vi "S4 Step Run For Scan.vi"(8 "error in (no error)":errorcluster) -> (0 "error out":errorcluster)   [LabVIEW 2019]
uses:
  NG Pick/NG Pick.lvclass
  Ctrl/Station Action.ctl
  Ctrl/ProjectStepSelect.ctl
  Ctrl/StationCmdSelect.ctl
  Ctrl/Auto Inspection Station Name2.ctl
  Ctrl/Auto Inspection Data Name.ctl
  Ctrl/S2 Station IO.ctl
  Global/Process Global.vi
  LineScan/LineScan.lvclass
  Ctrl/MeasureDisplayTab.ctl
  Ctrl/Table Save.ctl
  LLB/Commonly VI/Main Glb.vi
  LLB/Commonly VI.lvlib
panel:
  in  "Table Control":string[][](table)=[["PCBA BARCODE", ""], ["硬體(Tool初始化)", ""], ["company(Tool初始化)", ""], ["耗電流 uA(電流表)", "T"], ["電池負載電壓", "T"], ["晶片ID(Tool FORMAT)", "F"], ["雷雕ID(TOOl scan、藍芽接收器)", "S"], ["Format(Tool FORMAT)", "F"], ["Programe(Tool Programe)", "P"]]
  out "Numeric":dbl
  out "subarray":string[](array[string])
  out "S2 receive":string
  out "Blue Scan2 receive":string
  out "S1 receive":string
  out "S1 ToolStringOut":string
  out "S1 ChkSum":string
  out "Blue Scan receive":string
  out "Array":string[](array[string])
  out "present":i32
  out "Retry":i32
  out "Act Step":i32
  out "retry次數":string[](array[string])
  out "CurrentCmd":string
  out "Station Out":T1=enum."ImformOut"
  out "NG Pick out":refnum<class "NG Pick.lvclass">
  in  "NG Pick in":refnum<class "NG Pick.lvclass">
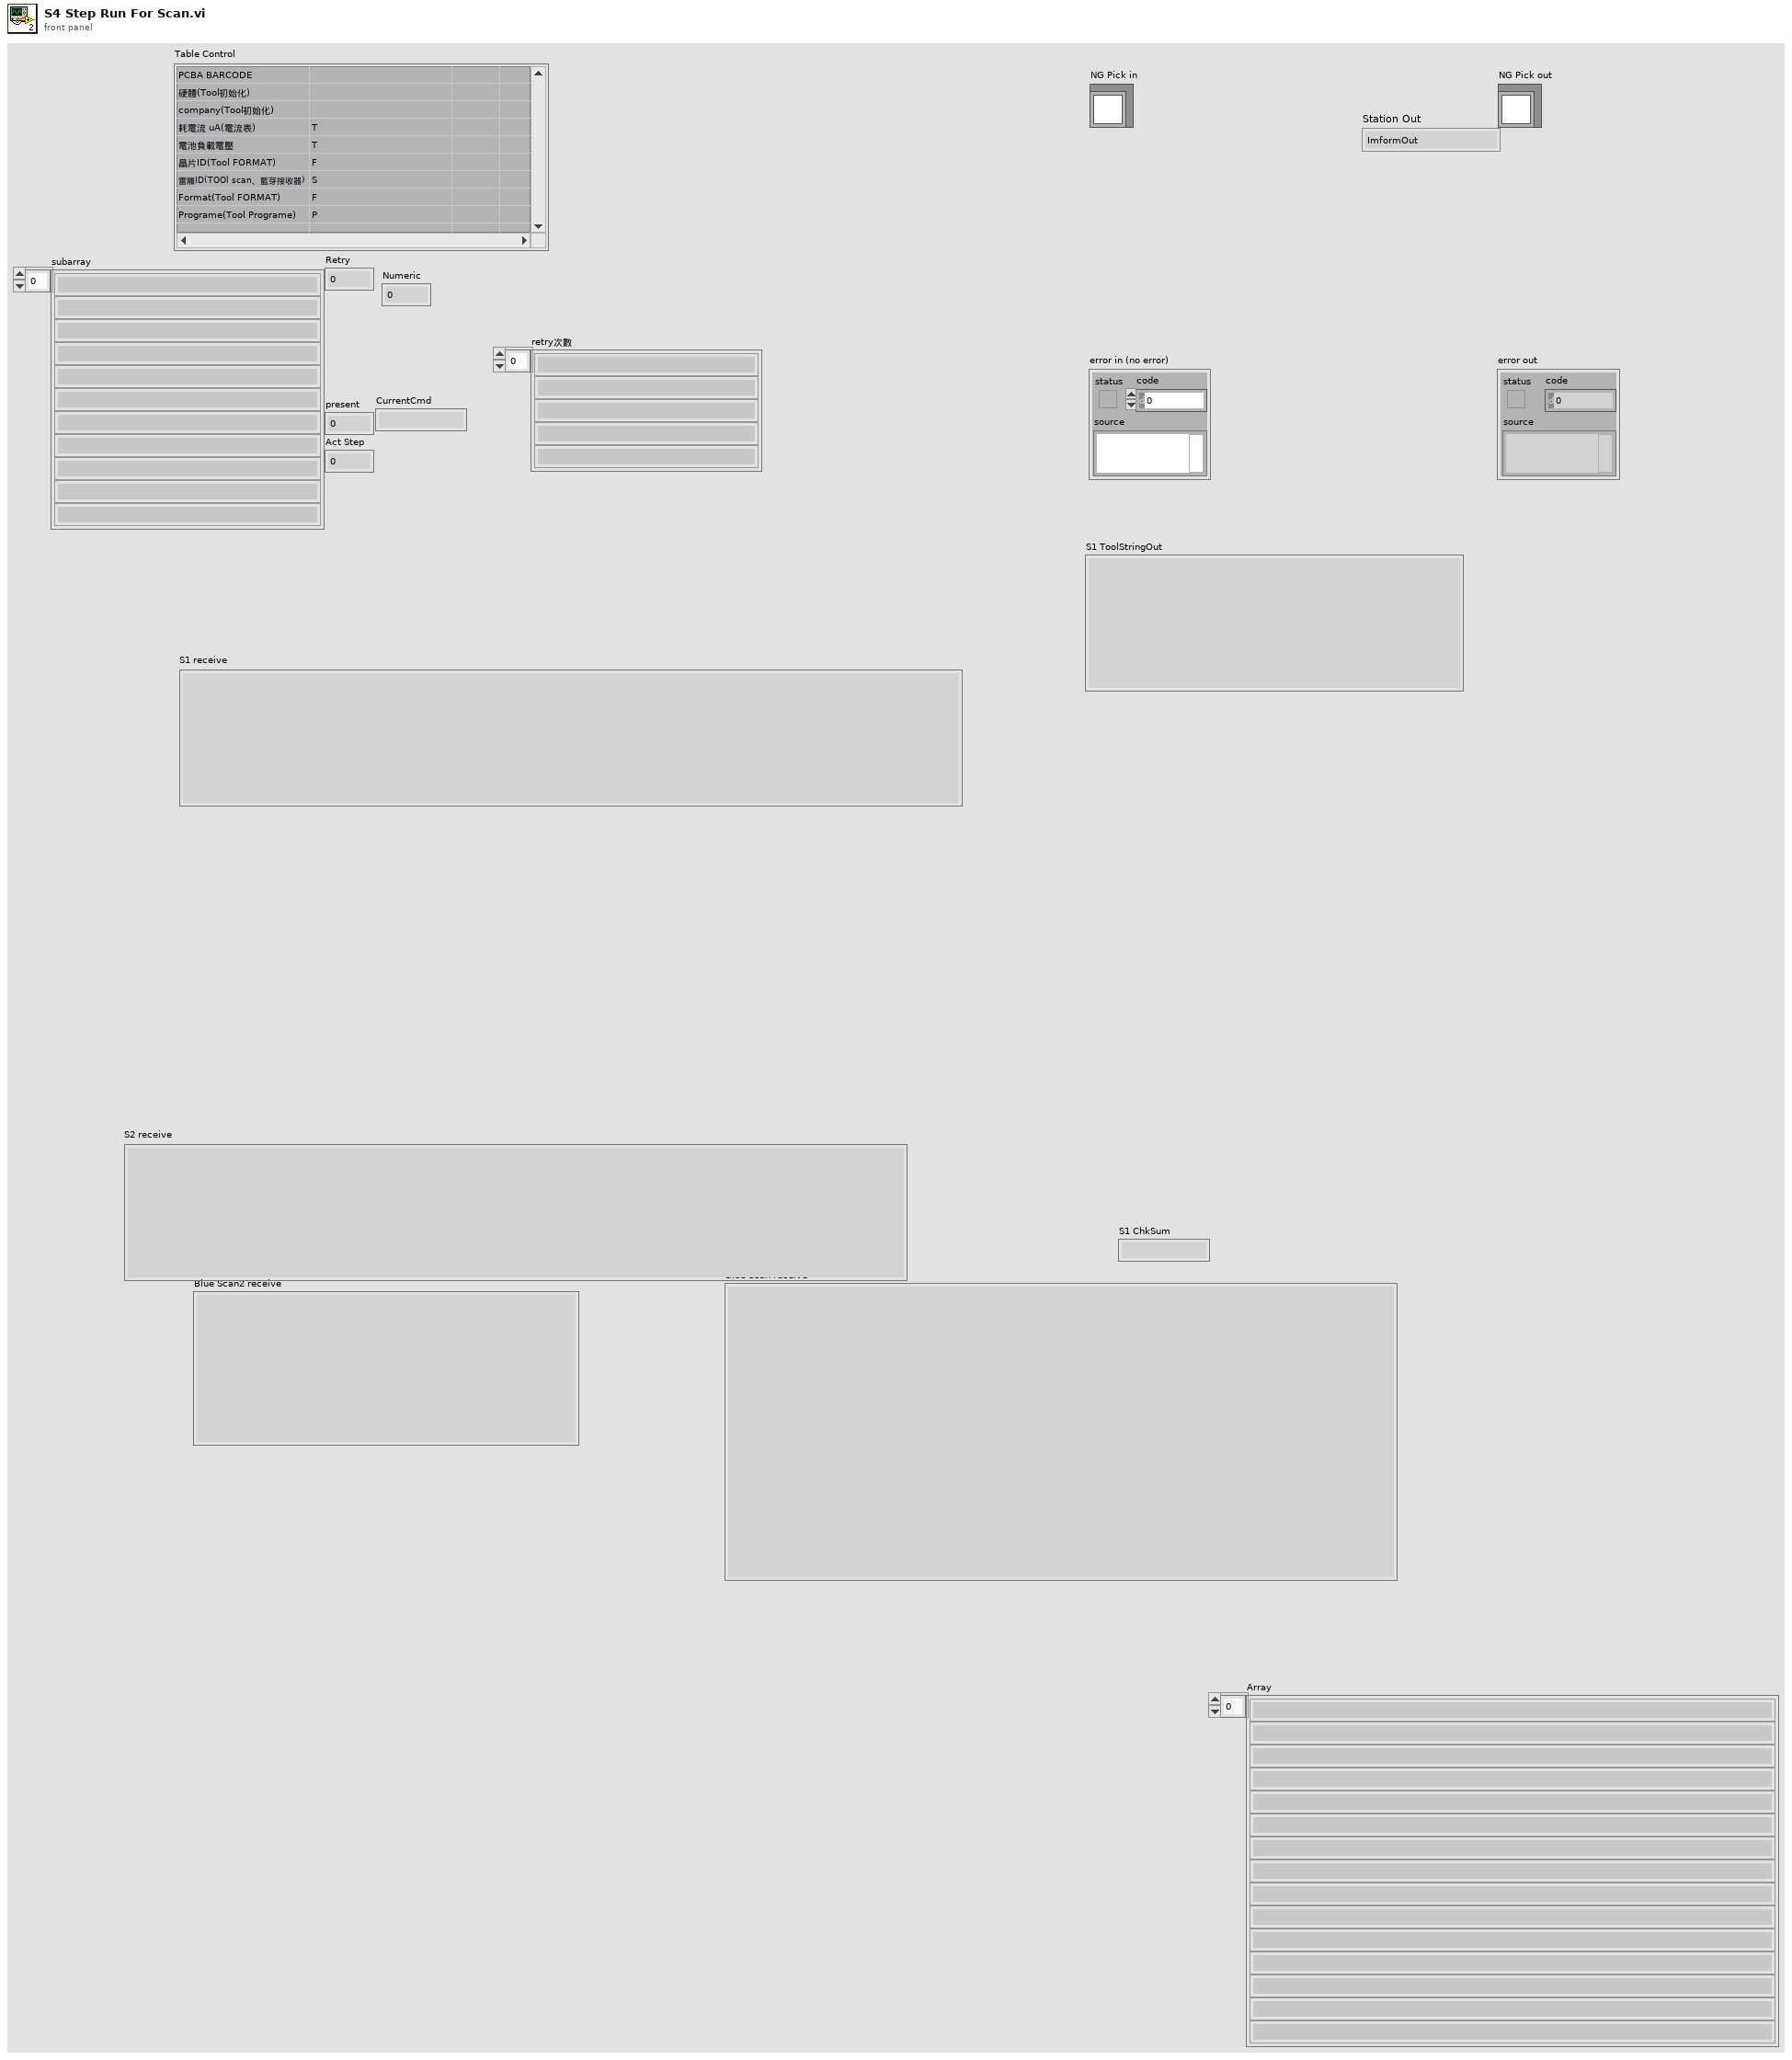
[diagram p1: front panel]
types:
  T1 = typedef "Station Action.ctl" = enum16{"Wait Item In", "Dectect Action", "ImformOut"}
  T2 = typedef "StationCmdSelect.ctl" = enum16{"Action", "Command", "Return", "DTime", "Retry"}
  T3 = typedef "Auto Inspection Data Name.ctl" = enum16{"LocalRun", "ItemSN(TimeCode)", "CurrentAction", "Error", "Data", "OKNG", "電壓值", "電壓值判斷", "電流值", "電流值判斷", "Laser1 Data", "Laser2 Data", "Laser OKNG", "StationNO"}
  T4 = typedef "Auto Inspection Station Name2.ctl" = enum16{"S1Barcode", "S2Measure", "S3Measure", "S4Measure", "S5Measure", "S11_LaserCheck", "S8_Vision AI"}
  T5 = typedef "Table Save.ctl" = enum16{"initial", "Add", "Write", "Replace", "Delete", "REad", "RedTable", "Load"}
  T6 = typedef "MeasureDisplayTab.ctl" = enum16{"Tray Barcode", "PCBA BARCODE", "硬體(Tool初始化)", "company(Tool初始化)", "耗電流 uA(電流表)", "電池負載電壓", "晶片ID(Tool FORMAT)", "雷雕ID(TOOl scan、藍芽接收器)", "Format(Tool FORMAT)", "Programe(Tool Programe)", "MAC(藍芽接收器)", "ID(藍芽接收器)", "KPA(藍芽接收器)", "溫度(藍芽接收器)", "SENSOR電池電壓(藍芽接收器)", "RSSI(藍芽接收器)", "SensorType_315(FSK scan)", "FSKsnVol_315(FSK scan)", "FSKscanl_315(FSK scan)", "P_315(FSK scan)", "T_315(FSK scan)", "SensorType_433(ASK scan)", "ASKsnVol_433(ASK scan)", "ASKscan_433(ASK scan)", "P_433(ASK scan)", "T_433(ASK scan)", "測高Data"}
  T7 = typedef "ProjectStepSelect.ctl" = enum16{"ProjectName", "Name", "Initial", "Reset", "Format", "Program1", "Program2", "Scan", "Finish", "MToolWork", "DataCheck", "DataSave", "OutputPLC", "WaitInputS1", "WaitInputOff"}
  T8 = typedef "S2 Station IO.ctl" = enum16{"S2站PC動作中_20", "電流量測完成產品OK_21", "電流量測完成產品NG_22", "S2站Format 執行_23", "S2 Format OK_24", "S2 Format NG_25", "S2站燒入執行_26", "S2站燒入OK_27", "S2站燒入NG_28", "S2站動作完成_29", "S3 PC動作中_30", "S3 Format 此站執行_31", "S3 Format OK_32", "S3 Format NG_33", "S3 燒入程式 此站執行_34", "S3 燒入程式 OK_35", "S3 燒入程式 NG_36", "S3 備用_37", "S3 備用_38", "S3 動作完成_39", "S4 PC動作中_40", "S4 量測完成 產品正常_41", "S4 量測完成 產品NG_42", "S4 Format 此站執行_43", "S4 Format OK_44", "S4 Format NG_45", "S4 燒入 此站不執行_46", "S4 燒入程式 OK_47", "S4 燒入程式 NG_48", "S4 藍芽Scan OK_49", "S4 藍芽Scan NG_50", "S4 動作完成_51", "給PLC要量電流訊號", "給PLC要量電壓訊號"}
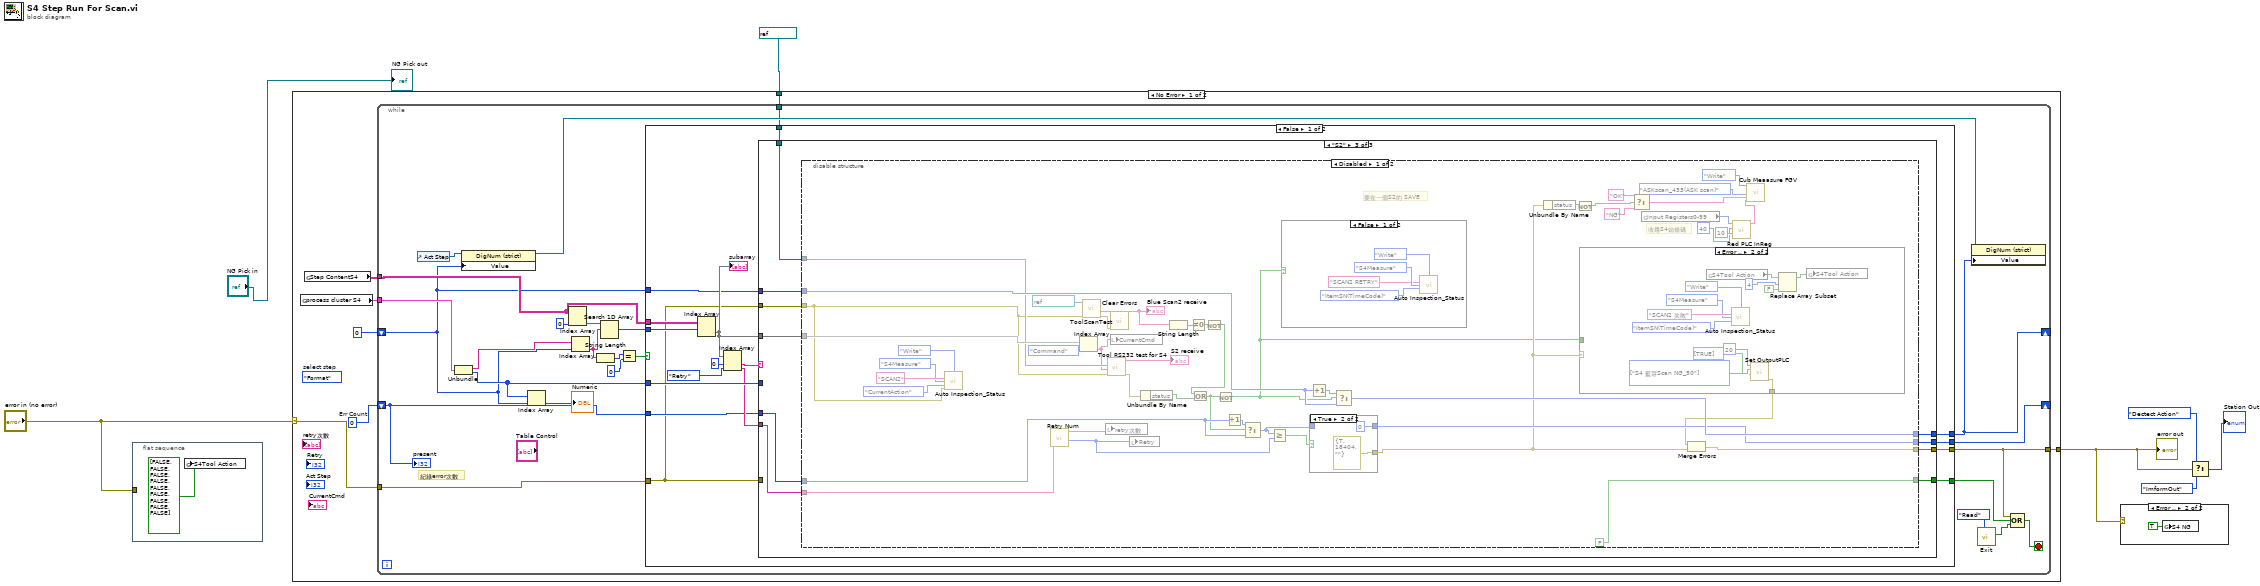
[diagram p0: block diagram]
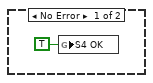
[diagram p2: hidden frame]
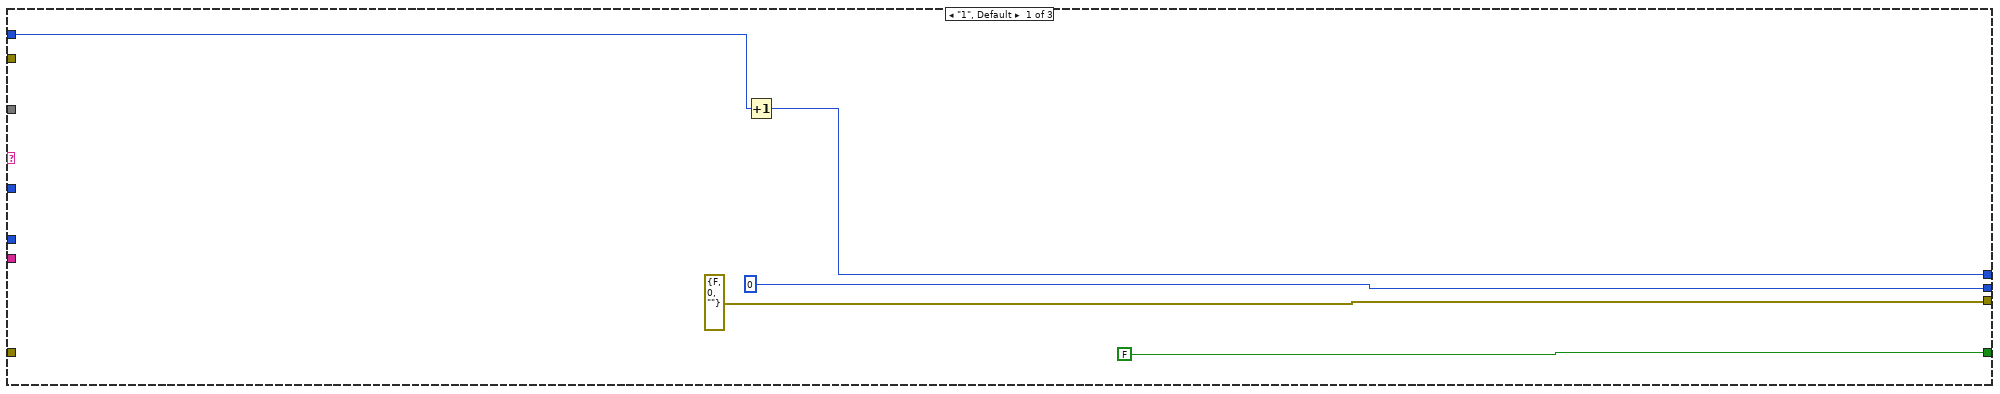
[diagram p3: hidden frame]
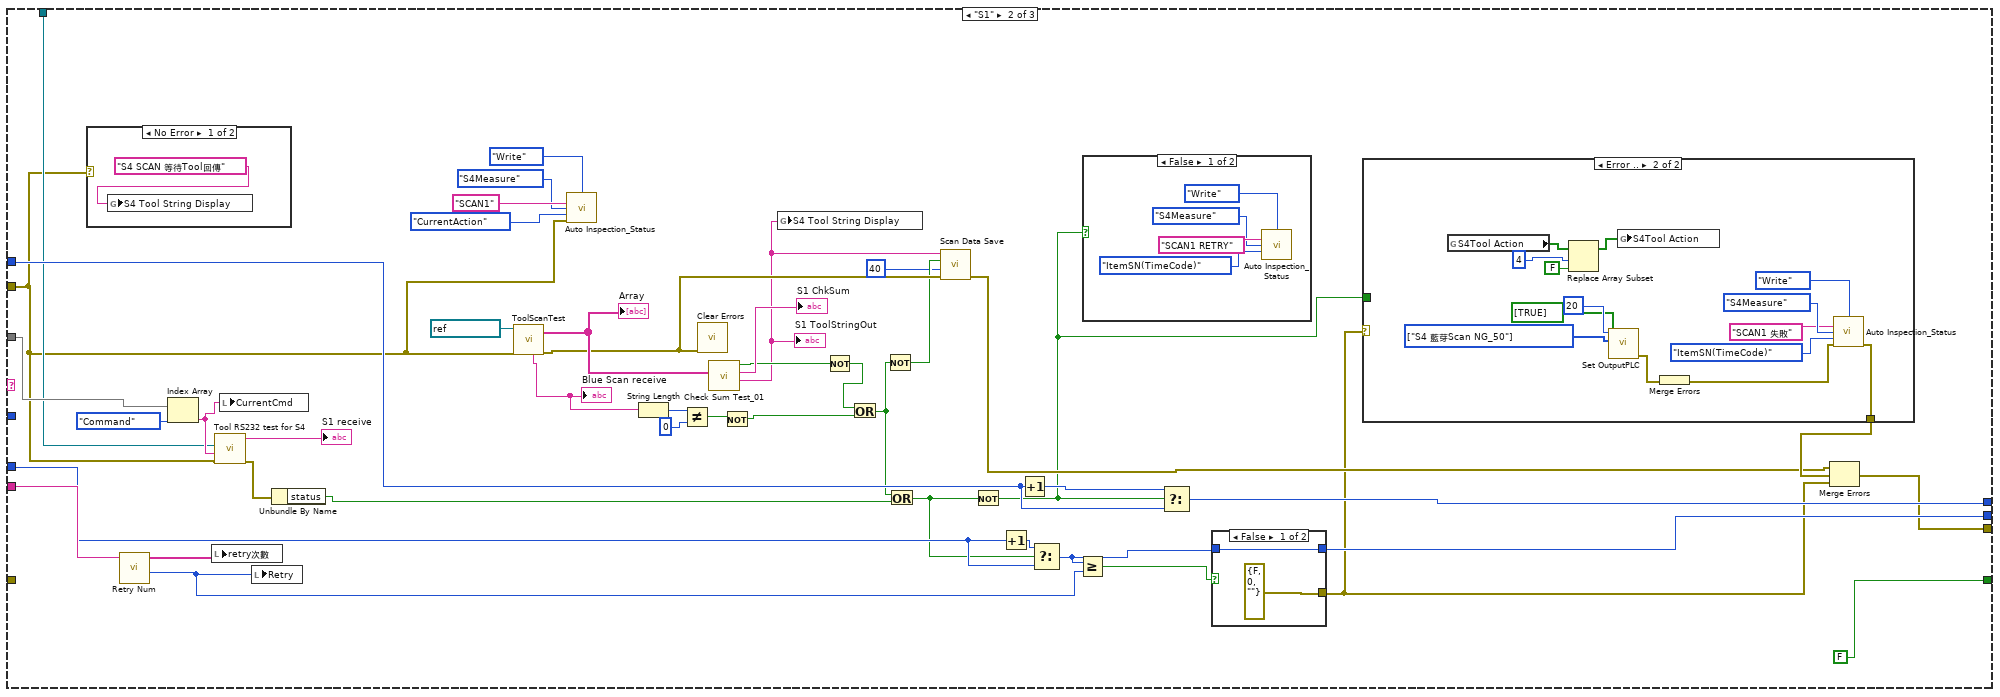
[diagram p4: hidden frame]
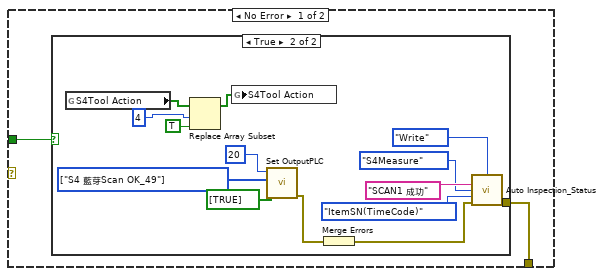
[diagram p7: hidden frame]
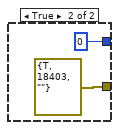
[diagram p9: hidden frame]
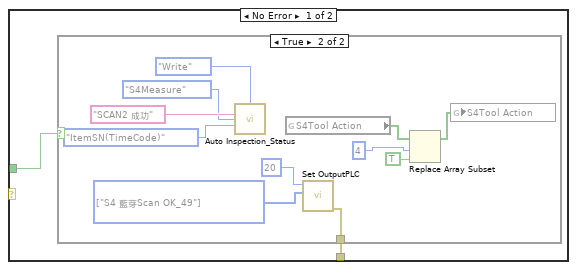
[diagram p11: hidden frame]
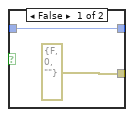
[diagram p13: hidden frame]
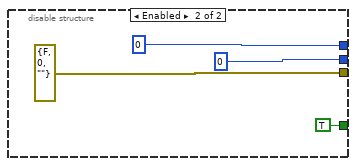
[diagram p14: hidden frame]
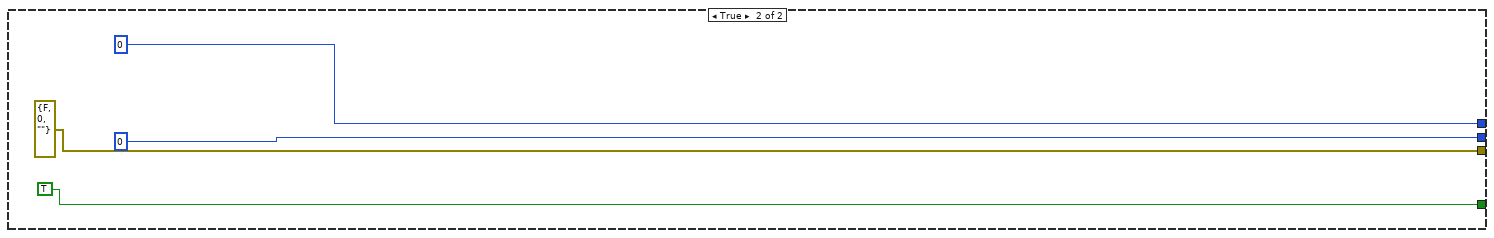
[diagram p15: hidden frame]
diagram:
  n1 = flat-sequence {
    tunnel: "error in (no error)" -> [_]
    frame #0 {
      n2 = global write "Process Global.vi" "S4Tool Action"(bool[] [FALSE, FALSE, FALSE, FALSE, FALSE, FALSE, FALSE, FALSE, FALSE] ("S4Tool Action")) -> ()
    }
  }
  n3 = case shown="No Error" "error in (no error)" {
    selector: "error in (no error)" -> [w10 w243]
    tunnel: [w15 w243] -> w2
    tunnel: refnum<visa-resource-name> "COM2" ("VISA resource name") -> [w9 _]
    frame No Error {
      w11 = 0  # Err Count
      (unwired) ProjectStepSelect."Format"  # select step
      n4 = global read "Process Global.vi" "process cluster S4"() -> (w13:cluster{string[], i32[]})
      n5 = global read "Process Global.vi" "Step ContentS4"() -> (w14:string[][])
      n6 = while {
        tunnel: [w26] -> w15
        shift-right: [w21] -> _
        shift-left: 0 -> [w22]
        shift-right: [w24] -> _
        shift-left: w11 -> [w25]
        tunnel: w14 -> [w37]
        tunnel: w13 -> [w36]
        tunnel: w10 -> [w19]
        tunnel: w9 -> [w18]
        stop <- w38 stop-if-true
        # "紀錄error次數"
        n7 = control-ref of="Act Step"() -> (w23:refnum<vi>)
        n8 = Unbundle(w36) -> (w39:string[], w40:i32[])
        n9 = property class="DigNum (strict)"(reference=w23, "Value"=w22) -> (reference out=w20:refnum<vi>)  [unwired: 1 in, 1 out]
        n10 = Index Array(array=w40, index=w22) -> (element=→"Numeric":i32)
        n11 = Index Array(array=w37, index (col)=0 ("disabled index (col)")) -> (element=w34:string[])  [unwired: 1 in]
        n12 = Index Array(array=w39, index=w22) -> (element=w30:string)
        n13 = String Length(string=w30) -> (length=w31:i32)
        n14 = Search 1D Array(1D array=w34, element=w30) -> (index of element=w33:i32)  [unwired: 1 in]
        n15 = Equal?(x=w31, y=0) -> (x = y?=w28:bool)
        n16 = case shown="False" w28 {
          tunnel: w40 -> [w56 _]
          tunnel: w37 -> [w55 _]
          tunnel: w33 -> [w54 _]
          tunnel: [w43 TRUE] -> w27
          tunnel: [w46 errorcluster {"status"=FALSE, "code"=0, "source"=""} ("error constant")] -> w26
          tunnel: w22 -> [w49 _]
          tunnel: [w48 0] -> w21
          tunnel: w25 -> [w47 _]
          tunnel: [w45 0 ("Err Count")] -> w24
          tunnel: w19 -> [w42 _]
          tunnel: w18 -> [w41 _]
          frame False {
            n17 = Index Array(array=w55, index (row)=w54) -> (element=w50:string[])  [unwired: 1 in]
            "subarray" <- w50
            n18 = Index Array(array=w50, index #1=0 ("index"), index #2=StationCmdSelect."Retry") -> (element #1=w52:string, element #2=w51:string)
            n19 = case shown="\"S2\"" w52 {
              tunnel: w56 -> [_ _ _]
              tunnel: w51 -> [_ w95 w152]
              tunnel: w50 -> [_ w94 w153]
              tunnel: w49 -> [w61 w93 w154]
              tunnel: [w60 w97 w150] -> w48
              tunnel: w47 -> [_ w92 w151]
              tunnel: [errorcluster {"status"=FALSE, "code"=0, "source"=""} ("error IO") w82 w148] -> w46
              tunnel: [0 ("Err Count") w96 w149] -> w45
              tunnel: [FALSE FALSE w155] -> w43
              tunnel: w42 -> [_ _ _]
              tunnel: w42 -> [_ w64 w146]
              tunnel: w41 -> [_ w83 w147]
              frame "1", Default {
                n20 = Increment(x=w61) -> (x+1=w60:i32)
              }
              frame "S1" {
                n21 = case shown="No Error" w64 {
                  frame No Error {
                    n22 = global write "Process Global.vi" "S4 Tool String Display"("S4 SCAN 等待Tool回傳") -> ()
                  }
                  frame Error {
                  }
                }
                n23 = call "Retry Num.vi"("String"=w95) -> ("Numeric"=w102:i32, "retry次數"=w99:string[])  [unwired: 9 in]
                n24 = Index Array(array=w94, index=StationCmdSelect."Command") -> (element=w91:string)
                n25 = local write "retry次數"(w99) -> ()
                n26 = call "Tool RS232 test for S4.vi"("error in (no error)"=w64, "Cmd In"=w91, "VISA resource name"=w83) -> ("error out"=w105:errorcluster, "receive string"=→"S1 receive":string)  [unwired: 7 in]
                n27 = local write "CurrentCmd"(w91) -> ()
                n28 = local write "Retry"(w102) -> ()
                n29 = Unbundle By Name(w105) -> ("status"=w89:bool)
                n30 = call "ToolScanTest.vi"("error in (no error)"=w64, "VISA resource name"=refnum<visa-resource-name> "COM10") -> ("error out"=w71:errorcluster, "read string 6"=w77:string, "Array"=w78:string[])  [unwired: 4 in, 3 out]
                "Blue Scan receive" <- w77
                "Array" <- w78
                n31 = call "Auto Inspection_Status.vi"("Action"=enum16{"Initial", "Write", "Read"}."Write", "DataIn"="SCAN1", "Station"=Auto_Inspection_Station_Name2."S4Measure", "Data"=Auto_Inspection_Data_Name."CurrentAction", "error in"=w64) -> ()  [unwired: 8 in, 3 out]
                n32 = String Length(string=w77) -> (length=w76:i32)
                n33 = Not Equal?(x=w76, y=0) -> (x != y?=w74:bool)
                n34 = call <vilib>:"Clear Errors.vi"("error in (no error)"=w71) -> ()  [unwired: 5 in, 2 out]
                n35 = call "Check Sum Test_01.vi"("Array"=w78) -> ("ToolStringOut_01"=w65:string, "ChkSum"=→"S1 ChkSum":string, "x = y?"=w80:bool)  [unwired: 8 in]
                "S1 ToolStringOut" <- w65
                n36 = Not(x=w74) -> (.not. x?=w73:bool)
                n37 = global write "Process Global.vi" "S4 Tool String Display"(w65) -> ()
                n38 = Not(x=w80) -> (.not. x?=w70:bool)
                n39 = Or(x=w70, y=w73) -> (x .or. y?=w68:bool)
                n40 = Not(x=w68) -> (.not. x?=w67:bool)
                n41 = Or(x=w68, y=w89) -> (x .or. y?=w88:bool)
                n42 = call "Scan Data Save.vi"("error in (no error)"=w71, "index"=40, "OK and NG"=w67, "String In"=w65) -> ("error out"=w69:errorcluster)  [unwired: 7 in]
                n43 = Not(x=w88) -> (.not. x?=w62:bool)
                n44 = Increment(x=w92) -> (x+1=w103:i32)
                n45 = Increment(x=w93) -> (x+1=w104:i32)
                n46 = Select(t=w103, s=w88, f=w92) -> (s? t:f=w100:i32)
                n47 = Greater Or Equal?(x=w100, y=w102) -> (x >= y?=w101:bool)
                n48 = case shown="False" w62 {
                  frame False {
                    n49 = call "Auto Inspection_Status.vi"("Action"=enum16{"Initial", "Write", "Read"}."Write", "DataIn"="SCAN1 RETRY", "Station"=Auto_Inspection_Station_Name2."S4Measure", "Data"=Auto_Inspection_Data_Name."ItemSN(TimeCode)") -> ()  [unwired: 9 in, 3 out]
                  }
                  frame True {
                  }
                }
                n50 = Select(t=w104, s=w62, f=w93) -> (s? t:f=w97:i32)
                n51 = case shown="False" w101 {
                  tunnel: [errorcluster {"status"=FALSE, "code"=0, "source"=""} ("error constant") errorcluster {"status"=TRUE, "code"=18403, "source"=""} ("error constant")] -> w63
                  tunnel: w100 -> [w142 _]
                  tunnel: [w142 0] -> w96
                  frame False {
                  }
                  frame True {
                  }
                }
                n52 = case shown="Error .." w63 {
                  tunnel: [w113 w132] -> w72
                  tunnel: w62 -> [w112 _]
                  frame No Error {
                    n53 = case shown="True" w112 {
                      tunnel: [_ w119] -> w113
                      frame False {
                      }
                      frame True {
                        w126 = T8[] [enum."S4 藍芽Scan OK_49"] items=["S2站PC動作中_20", "電流量測完成產品OK_21", "電流量測完成產品NG_22", "S2站Format 執行_23", "S2 Format OK_24", "S2 Format NG_25", "S2站燒入執行_26", "S2站燒入OK_27", "S2站燒入NG_28", "S2站動作完成_29", "S3 PC動作中_30", "S3 Format 此站執行_31", "S3 Format OK_32", "S3 Format NG_33", "S3 燒入程式 此站執行_34", "S3 燒入程式 OK_35", "S3 燒入程式 NG_36", "S3 備用_37", "S3 備用_38", "S3 動作完成_39", "S4 PC動作中_40", "S4 量測完成 產品正常_41", "S4 量測完成 產品NG_42", "S4 Format 此站執行_43", "S4 Format OK_44", "S4 Format NG_45", "S4 燒入 此站不執行_46", "S4 燒入程式 OK_47", "S4 燒入程式 NG_48", "S4 藍芽Scan OK_49", "S4 藍芽Scan NG_50", "S4 動作完成_51", "給PLC要量電流訊號", "給PLC要量電壓訊號"]
                        n54 = global read "Process Global.vi" "S4Tool Action"() -> (w118:bool[])
                        n55 = Replace Array Subset(array=w118, new element=TRUE ("new element/subarray"), index=4) -> (w115:bool[])
                        n56 = global write "Process Global.vi" "S4Tool Action"(w115) -> ()
                        n57 = call "Set OutputPLC.vi"("Address In"=20, "Array 2"=w126, "Sat Coils"=bool[] [TRUE]) -> ("Error Out"=w121:errorcluster[])  [unwired: 7 in]
                        n58 = Merge Errors(w121) -> (w120:errorcluster)
                        n59 = call "Auto Inspection_Status.vi"("Action"=enum16{"Initial", "Write", "Read"}."Write", "DataIn"="SCAN1 成功", "Station"=Auto_Inspection_Station_Name2."S4Measure", "Data"=Auto_Inspection_Data_Name."ItemSN(TimeCode)", "error in"=w120) -> ("error out"=w119:errorcluster)  [unwired: 8 in, 2 out]
                      }
                    }
                  }
                  frame Error {
                    w141 = T8[] [enum."S4 藍芽Scan NG_50"] items=["S2站PC動作中_20", "電流量測完成產品OK_21", "電流量測完成產品NG_22", "S2站Format 執行_23", "S2 Format OK_24", "S2 Format NG_25", "S2站燒入執行_26", "S2站燒入OK_27", "S2站燒入NG_28", "S2站動作完成_29", "S3 PC動作中_30", "S3 Format 此站執行_31", "S3 Format OK_32", "S3 Format NG_33", "S3 燒入程式 此站執行_34", "S3 燒入程式 OK_35", "S3 燒入程式 NG_36", "S3 備用_37", "S3 備用_38", "S3 動作完成_39", "S4 PC動作中_40", "S4 量測完成 產品正常_41", "S4 量測完成 產品NG_42", "S4 Format 此站執行_43", "S4 Format OK_44", "S4 Format NG_45", "S4 燒入 此站不執行_46", "S4 燒入程式 OK_47", "S4 燒入程式 NG_48", "S4 藍芽Scan OK_49", "S4 藍芽Scan NG_50", "S4 動作完成_51", "給PLC要量電流訊號", "給PLC要量電壓訊號"]
                    n60 = global read "Process Global.vi" "S4Tool Action"() -> (w131:bool[])
                    n61 = Replace Array Subset(array=w131, new element=FALSE ("new element/subarray"), index=4) -> (w128:bool[])
                    n62 = call "Set OutputPLC.vi"("Address In"=20, "Array 2"=w141, "Sat Coils"=bool[] [TRUE]) -> ("Error Out"=w134:errorcluster[])  [unwired: 7 in]
                    n63 = global write "Process Global.vi" "S4Tool Action"(w128) -> ()
                    n64 = Merge Errors(w134) -> (w133:errorcluster)
                    n65 = call "Auto Inspection_Status.vi"("Action"=enum16{"Initial", "Write", "Read"}."Write", "DataIn"="SCAN1 失敗", "Station"=Auto_Inspection_Station_Name2."S4Measure", "Data"=Auto_Inspection_Data_Name."ItemSN(TimeCode)", "error in"=w133) -> ("error out"=w132:errorcluster)  [unwired: 8 in, 2 out]
                  }
                }
                n66 = Merge Errors(w69, w72, w63) -> (w82:errorcluster)
              }
              frame "S2" {
                n67 = disable-structure shown="Disabled" {
                  disable-tunnel: [FALSE TRUE] -> w155
                  disable-tunnel: w154 -> [w200 _]
                  disable-tunnel: w153 -> [w199 _]
                  disable-tunnel: w152 -> [w198 _]
                  disable-tunnel: w151 -> [w197 _]
                  disable-tunnel: [w196 0] -> w150
                  disable-tunnel: [w195 0 ("Err Count")] -> w149
                  disable-tunnel: [w194 errorcluster {"status"=FALSE, "code"=0, "source"=""} ("error IO")] -> w148
                  disable-tunnel: w147 -> [w193 _]
                  disable-tunnel: w146 -> [w157 _]
                  frame Disabled {
                    # "要在一個S2的 SAVE"
                    # "收尋S4站條碼"
                    n68 = call "Auto Inspection_Status.vi"("Action"=enum16{"Initial", "Write", "Read"}."Write", "DataIn"="SCAN2", "Station"=Auto_Inspection_Station_Name2."S4Measure", "Data"=Auto_Inspection_Data_Name."CurrentAction", "error in"=w157) -> ()  [unwired: 8 in, 3 out]
                    n69 = call "Retry Num.vi"("String"=w198) -> ("Numeric"=w188:i32, "retry次數"=w185:string[])  [unwired: 9 in]
                    n70 = Index Array(array=w199, index=StationCmdSelect."Command") -> (element=w184:string)
                    n71 = call "ToolScanTest.vi"("error in (no error)"=w157, "VISA resource name"=refnum<visa-resource-name> "COM10") -> ("error out"=w183:errorcluster, "read string 3"=w181:string)  [unwired: 4 in, 4 out]
                    "Blue Scan2 receive" <- w181
                    n72 = local write "retry次數"(w185) -> ()
                    n73 = call "Tool RS232 test for S4.vi"("error in (no error)"=w157, "Cmd In"=w184, "VISA resource name"=w193) -> ("error out"=w191:errorcluster, "receive string"=→"S2 receive":string)  [unwired: 7 in]
                    n74 = local write "CurrentCmd"(w184) -> ()
                    n75 = call <vilib>:"Clear Errors.vi"("error in (no error)"=w183) -> ()  [unwired: 5 in, 2 out]
                    n76 = local write "Retry"(w188) -> ()
                    n77 = Unbundle By Name(w191) -> ("status"=w178:bool)
                    n78 = String Length(string=w181) -> (length=w182:i32)
                    n79 = Not Equal To 0?(x=w182) -> (x != 0?=w180:bool)
                    n80 = Not(x=w180) -> (.not. x?=w179:bool)
                    n81 = Or(x=w179, y=w178) -> (x .or. y?=w177:bool)
                    n82 = Not(x=w177) -> (.not. x?=w156:bool)
                    n83 = Increment(x=w197) -> (x+1=w189:i32)
                    n84 = Select(t=w189, s=w177, f=w197) -> (s? t:f=w186:i32)
                    n85 = Greater Or Equal?(x=w186, y=w188) -> (x >= y?=w187:bool)
                    n86 = case shown="False" w156 {
                      frame False {
                        n87 = call "Auto Inspection_Status.vi"("Action"=enum16{"Initial", "Write", "Read"}."Write", "DataIn"="SCAN2 RETRY", "Station"=Auto_Inspection_Station_Name2."S4Measure", "Data"=Auto_Inspection_Data_Name."ItemSN(TimeCode)") -> ()  [unwired: 9 in, 3 out]
                      }
                      frame True {
                      }
                    }
                    n88 = case shown="True" w187 {
                      tunnel: [errorcluster {"status"=FALSE, "code"=0, "source"=""} ("error constant") errorcluster {"status"=TRUE, "code"=18404, "source"=""} ("error constant")] -> w162
                      tunnel: w186 -> [w231 _]
                      tunnel: [w231 0] -> w195
                      frame False {
                      }
                      frame True {
                      }
                    }
                    n89 = Increment(x=w200) -> (x+1=w190:i32)
                    n90 = Select(t=w190, s=w156, f=w200) -> (s? t:f=w196:i32)
                    n91 = Unbundle By Name(w162) -> ("status"=w164:bool)
                    n92 = Not(x=w164) -> (.not. x?=w163:bool)
                    n93 = case shown="Error .." w162 {
                      tunnel: [w207 w228] -> w174
                      tunnel: w156 -> [w206 _]
                      frame No Error {
                        n94 = case shown="True" w206 {
                          tunnel: [_ w217] -> w207
                          frame False {
                          }
                          frame True {
                            w216 = T8[] [enum."S4 藍芽Scan OK_49"] items=["S2站PC動作中_20", "電流量測完成產品OK_21", "電流量測完成產品NG_22", "S2站Format 執行_23", "S2 Format OK_24", "S2 Format NG_25", "S2站燒入執行_26", "S2站燒入OK_27", "S2站燒入NG_28", "S2站動作完成_29", "S3 PC動作中_30", "S3 Format 此站執行_31", "S3 Format OK_32", "S3 Format NG_33", "S3 燒入程式 此站執行_34", "S3 燒入程式 OK_35", "S3 燒入程式 NG_36", "S3 備用_37", "S3 備用_38", "S3 動作完成_39", "S4 PC動作中_40", "S4 量測完成 產品正常_41", "S4 量測完成 產品NG_42", "S4 Format 此站執行_43", "S4 Format OK_44", "S4 Format NG_45", "S4 燒入 此站不執行_46", "S4 燒入程式 OK_47", "S4 燒入程式 NG_48", "S4 藍芽Scan OK_49", "S4 藍芽Scan NG_50", "S4 動作完成_51", "給PLC要量電流訊號", "給PLC要量電壓訊號"]
                            n95 = call "Auto Inspection_Status.vi"("Action"=enum16{"Initial", "Write", "Read"}."Write", "DataIn"="SCAN2 成功", "Station"=Auto_Inspection_Station_Name2."S4Measure", "Data"=Auto_Inspection_Data_Name."ItemSN(TimeCode)") -> ()  [unwired: 9 in, 3 out]
                            n96 = global read "Process Global.vi" "S4Tool Action"() -> (w215:bool[])
                            n97 = call "Set OutputPLC.vi"("Address In"=20, "Array 2"=w216) -> ("Error Out"=w217:errorcluster[])  [unwired: 8 in]
                            n98 = Replace Array Subset(array=w215, new element=TRUE ("new element/subarray"), index=4) -> (w208:bool[])
                            n99 = global write "Process Global.vi" "S4Tool Action"(w208) -> ()
                          }
                        }
                      }
                      frame Error {
                        w230 = T8[] [enum."S4 藍芽Scan NG_50"] items=["S2站PC動作中_20", "電流量測完成產品OK_21", "電流量測完成產品NG_22", "S2站Format 執行_23", "S2 Format OK_24", "S2 Format NG_25", "S2站燒入執行_26", "S2站燒入OK_27", "S2站燒入NG_28", "S2站動作完成_29", "S3 PC動作中_30", "S3 Format 此站執行_31", "S3 Format OK_32", "S3 Format NG_33", "S3 燒入程式 此站執行_34", "S3 燒入程式 OK_35", "S3 燒入程式 NG_36", "S3 備用_37", "S3 備用_38", "S3 動作完成_39", "S4 PC動作中_40", "S4 量測完成 產品正常_41", "S4 量測完成 產品NG_42", "S4 Format 此站執行_43", "S4 Format OK_44", "S4 Format NG_45", "S4 燒入 此站不執行_46", "S4 燒入程式 OK_47", "S4 燒入程式 NG_48", "S4 藍芽Scan OK_49", "S4 藍芽Scan NG_50", "S4 動作完成_51", "給PLC要量電流訊號", "給PLC要量電壓訊號"]
                        n100 = global read "Process Global.vi" "S4Tool Action"() -> (w226:bool[])
                        n101 = call "Auto Inspection_Status.vi"("Action"=enum16{"Initial", "Write", "Read"}."Write", "DataIn"="SCAN2 失敗", "Station"=Auto_Inspection_Station_Name2."S4Measure", "Data"=Auto_Inspection_Data_Name."ItemSN(TimeCode)") -> ()  [unwired: 9 in, 3 out]
                        n102 = call "Set OutputPLC.vi"("Address In"=20, "Array 2"=w230, "Sat Coils"=bool[] [TRUE]) -> ("Error Out"=w228:errorcluster[])  [unwired: 7 in]
                        n103 = Replace Array Subset(array=w226, new element=FALSE ("new element/subarray"), index=4) -> (w219:bool[])
                        n104 = global write "Process Global.vi" "S4Tool Action"(w219) -> ()
                      }
                    }
                    n105 = Select(t="OK" ("DataIn"), s=w163, f="NG" ("DataIn")) -> (s? t:f=w173:string)
                    n106 = global read "Main Glb.vi" "Input Registers0-99"() -> (w166:u16[])
                    n107 = Merge Errors(w174, w162) -> (w194:errorcluster)
                    n108 = call "Red PLC InReg.vi"("length"=10, "index"=40, "Input Registers Arr"=w166) -> ("Rad In Reg"=w167:string)  [unwired: 7 in, 1 out]
                    n109 = call "Cub Meaasure FGV.vi"("Action"=Table_Save."Write" ("Enum"), "Save Index"=MeasureDisplayTab."ASKscan_433(ASK scan)", "DataIn"=w173, "SN"=w167) -> ()  [unwired: 8 in, 8 out]
                  }
                  frame Enabled {
                  }
                }
              }
            }
          }
          frame True {
          }
        }
        n110 = property class="DigNum (strict)"(reference=w20, "Value"=w21) -> ()  [unwired: 1 in, 2 out]
        n111 = call "Exit.vi"("Enum"=enum16{"Initial", "Read", "Write"}."Read") -> ("ExitOut"=w17:bool)  [unwired: 10 in]
        n112 = Compound Arithmetic op=OR(w26, w27, w17) -> (w38:bool)
        "present" <- w25
      }
    }
    frame Error {
    }
  }
  "error out" <- w2
  n113 = case shown="Error .." w2 {
    frame No Error {
      n114 = global write "Process Global.vi" "S4 OK"(TRUE ("S4 OK")) -> ()
    }
    frame Error {
      n115 = global write "Process Global.vi" "S4 NG"(TRUE ("S4 NG")) -> ()
    }
  }
  n116 = Select(t=Station_Action."Dectect Action" ("Station Out"), s=w2, f=Station_Action."ImformOut" ("Station Out")) -> (s? t:f=→"Station Out":T1)
  "NG Pick out" <- "NG Pick in"
